vi "SocketHandle.vi"(0 "Socket in":refnum<class "TCPAlerts.lvclass">, 2 "Mode":enum16{"Open", "Read", "Write", "Close"}(ring), 7 "data in":string, 11 "error in (no error)":errorcluster) -> (4 "Socket out":refnum<class "TCPAlerts.lvclass">, 8 "data out":string, 15 "error out":errorcluster)   [LabVIEW 2011, in "TCPAlerts.lvclass"]
uses:
  TCPAlerts.lvclass
  TCPAlerts.lvclass/TCPAlerts.ctl
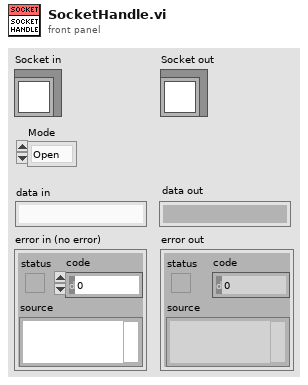
[diagram p1: front panel]
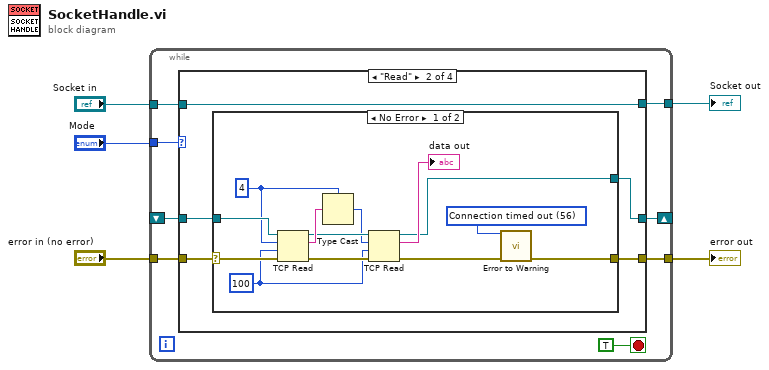
[diagram p0: block diagram]
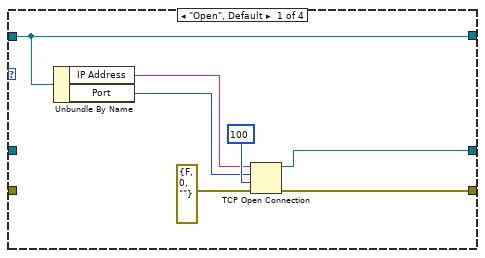
[diagram p2: hidden frame]
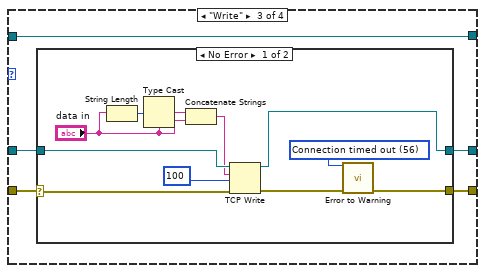
[diagram p4: hidden frame]
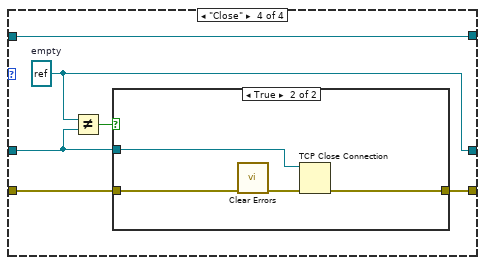
[diagram p6: hidden frame]
diagram:
  n1 = while {
    shift-right: [w13] -> _
    shift-left: _ -> [w10]
    tunnel: "Mode" -> [w9]
    tunnel: "error in (no error)" -> [w11]
    tunnel: [w12] -> w1
    tunnel: "Socket in" -> [w7]
    tunnel: [w6] -> w4
    stop <- TRUE stop-if-true
    n2 = case shown="\"Read\"" w9 {
      tunnel: [w19 w24 w44 w61] -> w13
      tunnel: [w17 w22 w43 w64] -> w12
      tunnel: w11 -> [_ w23 w42 w63]
      tunnel: w10 -> [_ w25 w45 w60]
      tunnel: w7 -> [w16 w21 w41 w59]
      tunnel: [w16 w21 w41 w59] -> w6
      frame "Open", Default {
        n3 = Unbundle By Name(w16) -> ("IP Address"=w15:string, "Port"=w14:u16)
        n4 = TCP Open Connection(address=w15, remote port or service name=w14, timeout ms (60000)=100, error in (no error)=errorcluster {"status"=FALSE, "code"=0, "source"=""} ("error constant")) -> (connection ID=w19:refnum<k5>, error out=w17:errorcluster)  [unwired: 1 out]
      }
      frame "Read" {
        n5 = case shown="No Error" w23 {
          selector: w23 -> [w37 w39]
          tunnel: w25 -> [w38 w40]
          tunnel: [w28 w40] -> w24
          tunnel: [w36 w39] -> w22
          frame No Error {
            w26 = 56 items=["No Error", "Argument Error", "Memory Full", "Out of Zone", "End of File", "File Already Open", "Generic File IO Error", "File Not Found", "File Permission Error", "Disk Full", "Duplicate Path", "Too Many Files Open", "Not Enabled", "Resource File Not Found", "Cannot Add Resource", "Resource Not Found", "Image Not Found", "Image Memory Error", "Pen Does Not Exist", "Config Bad Type", "Config Token Not Found", "Config Parse Error", "Config Memory Error", "Bad External Code Format", "Bad External Code Offset", "External Code Not Present", "Null Window", "Destroy Window Mixup", "Null Menu", "Print Aborted", "Bad Print Record", "Print Driver Error", "Windows Error During Print", "Memory Error During Print", "Print Dialog Error", "Generic Print Error", "Invalid Device Refnum", "Device Not Found", "Device Parameter Error", "Device Unit Error", "Can't Open Device", "Device Call Aborted", "Generic Error", "Cancelled By User", "Object ID Too Low", "Object ID Too High", "Object Not In Heap", "Unknown Heap", "Bad DefProc ID", "DefProc Not In Table", "Message Out Of Range", "Null Method", "Unknown Message", "Manager Call Not Supported", "Bad address", "Connection In progress", "Connection timed out", "Connection is already in progress", "Network attribute not supported", "Network error", "Address in use", "System out of memory", "Connection aborted", "Connection refused", "Connection is not connected", "Connection is already connected", "Connection closed", "Initialize error (interapplication manager)", "Bad occurrence", "Wait on unbound occurrence handler", "Occurrence queue overflow", "Bad path", "Semaphore not signaled", "Unrecognized type (interapplication manager)"] ("1st Error to Convert")
            w30 = 100
            w31 = 4 ("bytes to read")
            n6 = TCP Read(connection ID=w38, bytes to read=w31, error in (no error)=w37, 9:w30) -> (connection ID out=w33:refnum<k5>, data out=w34:string, error out=w35:errorcluster)  [unwired: 1 out]
            n7 = Type Cast(type=w31, x=w34) -> (*(type *) &x=w32:i32)
            n8 = TCP Read(connection ID=w33, bytes to read=w32, error in (no error)=w35, 9:w30) -> (connection ID out=w28:refnum<k5>, data out=→"data out":string, error out=w27:errorcluster)  [unwired: 1 out]
            n9 = call <vilib>:"Error to Warning.vi"("1st Error to Convert"=w26, "error in"=w27) -> ("warning out"=w36:errorcluster)  [unwired: 3 in, 10 out]
          }
          frame Error {
          }
        }
      }
      frame "Write" {
        n10 = case shown="No Error" w42 {
          selector: w42 -> [w53 w57]
          tunnel: w45 -> [w56 w58]
          tunnel: [w47 w58] -> w44
          tunnel: [w54 w57] -> w43
          frame No Error {
            w46 = 56 items=["No Error", "Argument Error", "Memory Full", "Out of Zone", "End of File", "File Already Open", "Generic File IO Error", "File Not Found", "File Permission Error", "Disk Full", "Duplicate Path", "Too Many Files Open", "Not Enabled", "Resource File Not Found", "Cannot Add Resource", "Resource Not Found", "Image Not Found", "Image Memory Error", "Pen Does Not Exist", "Config Bad Type", "Config Token Not Found", "Config Parse Error", "Config Memory Error", "Bad External Code Format", "Bad External Code Offset", "External Code Not Present", "Null Window", "Destroy Window Mixup", "Null Menu", "Print Aborted", "Bad Print Record", "Print Driver Error", "Windows Error During Print", "Memory Error During Print", "Print Dialog Error", "Generic Print Error", "Invalid Device Refnum", "Device Not Found", "Device Parameter Error", "Device Unit Error", "Can't Open Device", "Device Call Aborted", "Generic Error", "Cancelled By User", "Object ID Too Low", "Object ID Too High", "Object Not In Heap", "Unknown Heap", "Bad DefProc ID", "DefProc Not In Table", "Message Out Of Range", "Null Method", "Unknown Message", "Manager Call Not Supported", "Bad address", "Connection In progress", "Connection timed out", "Connection is already in progress", "Network attribute not supported", "Network error", "Address in use", "System out of memory", "Connection aborted", "Connection refused", "Connection is not connected", "Connection is already connected", "Connection closed", "Initialize error (interapplication manager)", "Bad occurrence", "Wait on unbound occurrence handler", "Occurrence queue overflow", "Bad path", "Semaphore not signaled", "Unrecognized type (interapplication manager)"] ("1st Error to Convert")
            n11 = String Length(string="data in") -> (length=w51:i32)
            n12 = Type Cast(type="data in", x=w51) -> (*(type *) &x=w52:string)
            n13 = Concatenate Strings(w52, "data in") -> (w49:string)
            n14 = TCP Write(connection ID=w56, data in=w49, error in (no error)=w53, 9:100 ("timeout ms (25000)")) -> (connection ID out=w47:refnum<k5>, error out=w48:errorcluster)  [unwired: 1 out]
            n15 = call <vilib>:"Error to Warning.vi"("1st Error to Convert"=w46, "error in"=w48) -> ("warning out"=w54:errorcluster)  [unwired: 3 in, 10 out]
          }
          frame Error {
          }
        }
      }
      frame "Close" {
        w61 = refnum<k5> refnum  # empty
        n16 = Not Equal?(x=w61, y=w60) -> (x != y?=w62:bool)
        n17 = case shown="True" w62 {
          tunnel: [w65 w69] -> w64
          tunnel: w63 -> [w65 w68]
          tunnel: w60 -> [_ w66]
          frame False {
          }
          frame True {
            n18 = call <vilib>:"Clear Errors.vi"("error in (no error)"=w68) -> ("error out"=w67:errorcluster)  [unwired: 6 in]
            n19 = TCP Close Connection(connection ID=w66, error in (no error)=w67) -> (error out=w69:errorcluster)  [unwired: 2 out]
          }
        }
      }
    }
  }
  "error out" <- w1
  "Socket out" <- w4
